vi "Update State Data.vi"(8 "error in (no error)":errorcluster, 9 "Data":variant, 10 "Argument":string, 11 "State Data":T1={"Core"={"Current VI Reference"=refnum, "Close Panel on Exit?"=FALSE}, "FP Refs"={"VI Tree"=refnum, "Window Title"=refnum, "Same Title as VI?"=refnum, "VI Desc"=refnum, "Help Path"=refnum, "Help Tag"=refnum, "Help URL"=refnum, "Controls"=refnum, "VI Connector Pane"=refnum, "Path to VI"=refnum, "Inlined?"=refnum, "Allow Debugging?"=refnum, "Auto Error Handling?"=refnum, "Run When Opened?"=refnum, "Suspend When Called?"=refnum, "Reentrancy"=refnum, "Priority"=refnum, "Preferred Exec System"=refnum, "VI Type"=refnum, "Edit Icon"=refnum, "Add Copyright"=refnum, "Set all VIs"=refnum, "Help Used"=refnum}, "Current Path"=path "", "New Item Data"=[], "Saved Item Data"=[], "FP"={"Selected VI Data"=0, "Help Path"="", "Help Tag"="", "Help URL"="", "Help Type"=enum."Local Help File", "VI Desc"="", "Controls"=[], "Window Title"="", "Same Title?"=FALSE, "VI Tree Value"=""}, "Config Path"=path "", "Config"={"ItemsEdited"=0, "Copyright Path"=path "", "Copyright Delimiter"="", "Recent Folders"=[], "Recent Files"=[], "Recent Filters"=[], "Abbreviate Names?"=FALSE, "Format Bold Tags?"=FALSE, "Show ConPane Only?"=FALSE, "Show Top-Level Only?"=FALSE, "Confirm Save?"=FALSE, "Confirm Revert?"=FALSE, "Confirm Save All?"=FALSE, "Confirm Revert All?"=FALSE, "Confirm Exit?"=FALSE, "Flat View?"=FALSE, "Ctls Sort Column"=0, "Ctls Sort Order"=0}, "Desc Selection"={"Selection Start"=0, "Selection End"=0}, "Displayed Indices"=[], "Filter"={"Filter Column"=enum."Description", "Filter Type"=enum."Contains", "Filter Value"="", "New Data?"=FALSE, "Case Sensitive?"=FALSE, "Enabled?"=FALSE}, "Sort"={"Sort Column"=enum."Description", "Ascending?"=FALSE, "Enabled?"=FALSE}, "Tree Map"=refnum, "Last Save Count"=0, "View Saved?"=FALSE, "Selected Item"=refnum}) -> (0 "error out":errorcluster, 3 "State Data out":T1={"Core"={"Current VI Reference"=refnum, "Close Panel on Exit?"=FALSE}, "FP Refs"={"VI Tree"=refnum, "Window Title"=refnum, "Same Title as VI?"=refnum, "VI Desc"=refnum, "Help Path"=refnum, "Help Tag"=refnum, "Help URL"=refnum, "Controls"=refnum, "VI Connector Pane"=refnum, "Path to VI"=refnum, "Inlined?"=refnum, "Allow Debugging?"=refnum, "Auto Error Handling?"=refnum, "Run When Opened?"=refnum, "Suspend When Called?"=refnum, "Reentrancy"=refnum, "Priority"=refnum, "Preferred Exec System"=refnum, "VI Type"=refnum, "Edit Icon"=refnum, "Add Copyright"=refnum, "Set all VIs"=refnum, "Help Used"=refnum}, "Current Path"=path "", "New Item Data"=[], "Saved Item Data"=[], "FP"={"Selected VI Data"=0, "Help Path"="", "Help Tag"="", "Help URL"="", "Help Type"=enum."Local Help File", "VI Desc"="", "Controls"=[], "Window Title"="", "Same Title?"=FALSE, "VI Tree Value"=""}, "Config Path"=path "", "Config"={"ItemsEdited"=0, "Copyright Path"=path "", "Copyright Delimiter"="", "Recent Folders"=[], "Recent Files"=[], "Recent Filters"=[], "Abbreviate Names?"=FALSE, "Format Bold Tags?"=FALSE, "Show ConPane Only?"=FALSE, "Show Top-Level Only?"=FALSE, "Confirm Save?"=FALSE, "Confirm Revert?"=FALSE, "Confirm Save All?"=FALSE, "Confirm Revert All?"=FALSE, "Confirm Exit?"=FALSE, "Flat View?"=FALSE, "Ctls Sort Column"=0, "Ctls Sort Order"=0}, "Desc Selection"={"Selection Start"=0, "Selection End"=0}, "Displayed Indices"=[], "Filter"={"Filter Column"=enum."Description", "Filter Type"=enum."Contains", "Filter Value"="", "New Data?"=FALSE, "Case Sensitive?"=FALSE, "Enabled?"=FALSE}, "Sort"={"Sort Column"=enum."Description", "Ascending?"=FALSE, "Enabled?"=FALSE}, "Tree Map"=refnum, "Last Save Count"=0, "View Saved?"=FALSE, "Selected Item"=refnum})   [LabVIEW 2020, in "VI Properties Editor.lvlib"]
doc: "Updates one or more elements of <B>State Data</B> based on <B>Argument</B> and <B>Data</B>."
uses:
  VI Properties Editor.lvlib
  Classes/Tree Map/Project Tree Map.lvclass
  Classes/Item/Item.lvclass
  Classes/VI/VI.lvclass
  <vilib>/ErrorRing/Error Ring.xnode
  Classes/Control/Control.lvclass
  3573416a-ab14-40fa-8eb1-e5c23e8662a1.vi
  6c3ab29c-e086-46da-822f-1f7a3bdde8cc.vi
  CTLs/Filter Column.ctl
  CTLs/Filter Type.ctl
  c05ae38d-f8ec-456d-8819-95a6d1f6576e.vi
  CTLs/Sort Column.ctl
  <vilib>/Utility/error.llb/Error Cluster From Error Code.vi
  CTLs/Main Front Panel Controls.ctl
  CTLs/Config.ctl
  <vilib>/Utility/miscctls.llb/LVSelectionTypeDef.ctl
  CTLs/Filter Info.ctl
  CTLs/Main References.ctl
  CTLs/Main State Data.ctl
  CTLs/Sort Info.ctl
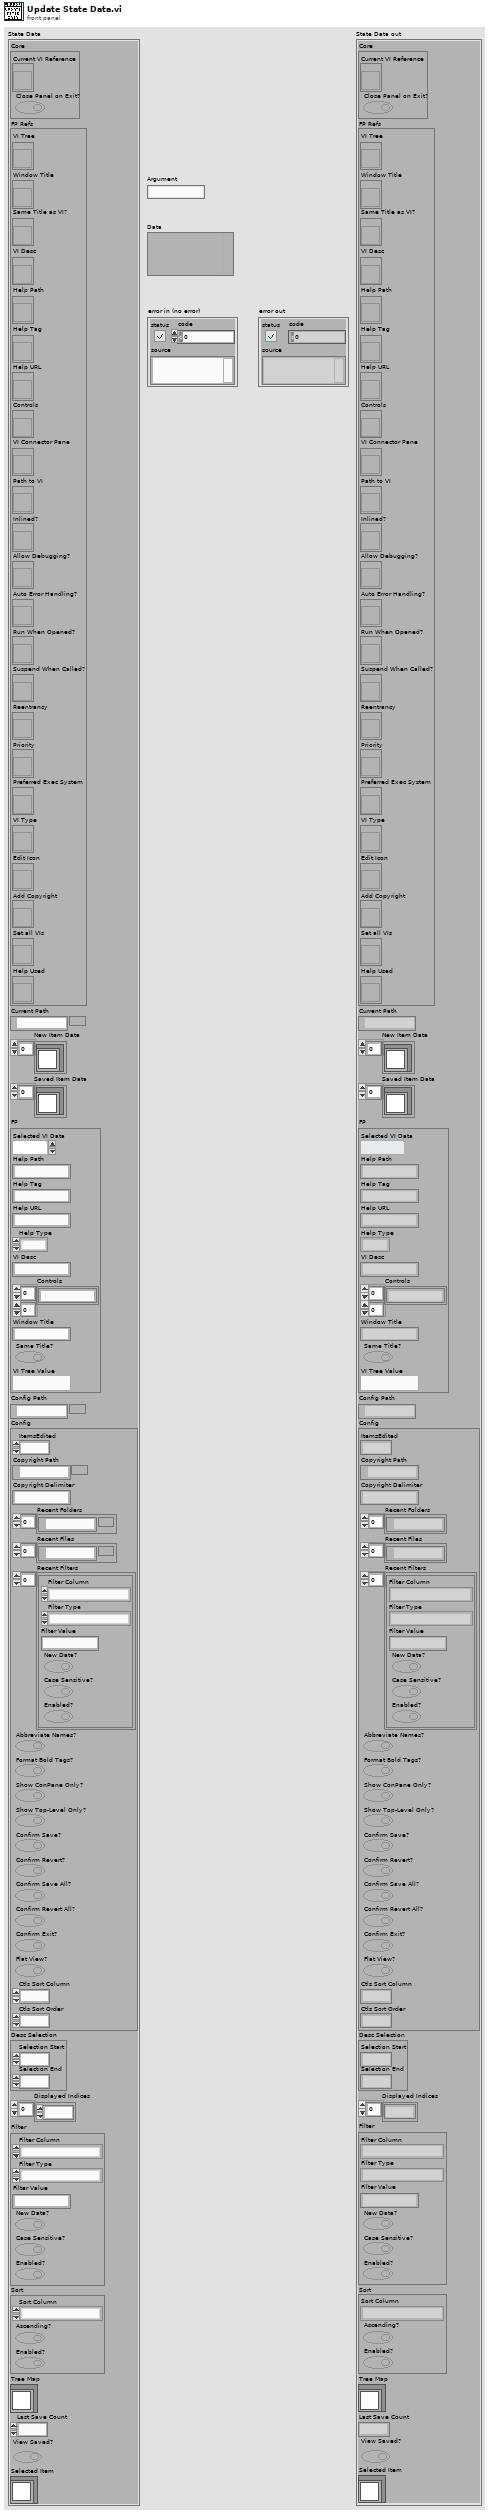
[diagram p1: front panel]
types:
  T1 = typedef "VI Properties Editor.lvlib/Main State Data.ctl" = cluster{"Core":cluster{"Current VI Reference":refnum<vi>, "Close Panel on Exit?":bool}, "FP Refs":T2, "Current Path":path, "New Item Data":refnum<class "Item.lvclass">[], "Saved Item Data":refnum<class "Item.lvclass">[], "FP":T3, "Config Path":path, "Config":T4, "Desc Selection":T8, "Displayed Indices":i32[], "Filter":T5, "Sort":T9, "Tree Map":refnum<class "Project Tree Map.lvclass">, "Last Save Count":u32, "View Saved?":bool, "Selected Item":refnum<class "Item.lvclass">}
  T2 = typedef "VI Properties Editor.lvlib/Main References.ctl" = cluster{"VI Tree":refnum<vi>, "Window Title":refnum<vi>, "Same Title as VI?":refnum<vi>, "VI Desc":refnum<vi>, "Help Path":refnum<vi>, "Help Tag":refnum<vi>, "Help URL":refnum<vi>, "Controls":refnum<vi>, "VI Connector Pane":refnum<vi>, "Path to VI":refnum<vi>, "Inlined?":refnum<vi>, "Allow Debugging?":refnum<vi>, "Auto Error Handling?":refnum<vi>, "Run When Opened?":refnum<vi>, "Suspend When Called?":refnum<vi>, "Reentrancy":refnum<vi>, "Priority":refnum<vi>, "Preferred Exec System":refnum<vi>, "VI Type":refnum<vi>, "Edit Icon":refnum<vi>, "Add Copyright":refnum<vi>, "Set all VIs":refnum<vi>, "Help Used":refnum<vi>}
  T3 = typedef "VI Properties Editor.lvlib/Main Front Panel Controls.ctl" = cluster{"Selected VI Data":i32, "Help Path":string, "Help Tag":string, "Help URL":string, "Help Type":enum16{"Local Help File", "Web-based Help"}, "VI Desc":string, "Controls":string[][], "Window Title":string, "Same Title?":bool, "VI Tree Value":string}
  T4 = typedef "VI Properties Editor.lvlib/Config.ctl" = cluster{"ItemsEdited":u32, "Copyright Path":path, "Copyright Delimiter":string, "Recent Folders":path[], "Recent Files":path[], "Recent Filters":T5[], "Abbreviate Names?":bool, "Format Bold Tags?":bool, "Show ConPane Only?":bool, "Show Top-Level Only?":bool, "Confirm Save?":bool, "Confirm Revert?":bool, "Confirm Save All?":bool, "Confirm Revert All?":bool, "Confirm Exit?":bool, "Flat View?":bool, "Ctls Sort Column":i32, "Ctls Sort Order":i32}
  T5 = typedef "VI Properties Editor.lvlib/Filter Info.ctl" = cluster{"Filter Column":T6, "Filter Type":T7, "Filter Value":string, "New Data?":bool, "Case Sensitive?":bool, "Enabled?":bool}
  T6 = typedef "VI Properties Editor.lvlib/Filter Column.ctl" = enum16{"Name", "Path", "Type", "Window Title", "Description", "Help Path", "Help Tag", "Custom Title?", "Reentrancy", "Inlined?", "Help URL", "Help Type", "Allow Debugging?", "Auto Error Handling?", "Run When Opened?", "Suspend When Called?", "Priority", "Preferred Exec Sytem", "Control Label", "Control Caption", "Control Description", "Control Tip Strip"}
  T7 = typedef "VI Properties Editor.lvlib/Filter Type.ctl" = enum16{"Contains", "Equals", "Starts with", "Ends with", "Is empty", "Does not contain", "Does not equal", "Is not empty"}
  T8 = typedef "LVSelectionTypeDef.ctl" = cluster{"Selection Start":u32, "Selection End":u32}
  T9 = typedef "VI Properties Editor.lvlib/Sort Info.ctl" = cluster{"Sort Column":T10, "Ascending?":bool, "Enabled?":bool}
  T10 = typedef "VI Properties Editor.lvlib/Sort Column.ctl" = enum16{"Name", "Filename", "Path", "Type", "Window Title", "Description", "Help Path", "Help Tag", "Custom Title?", "Reentrancy", "Inlined?", "Help URL", "Help Type", "Allow Debugging?", "Auto Error Handling?", "Run When Opened?", "Suspend When Called?", "Priority", "Preferred Exec Sytem"}
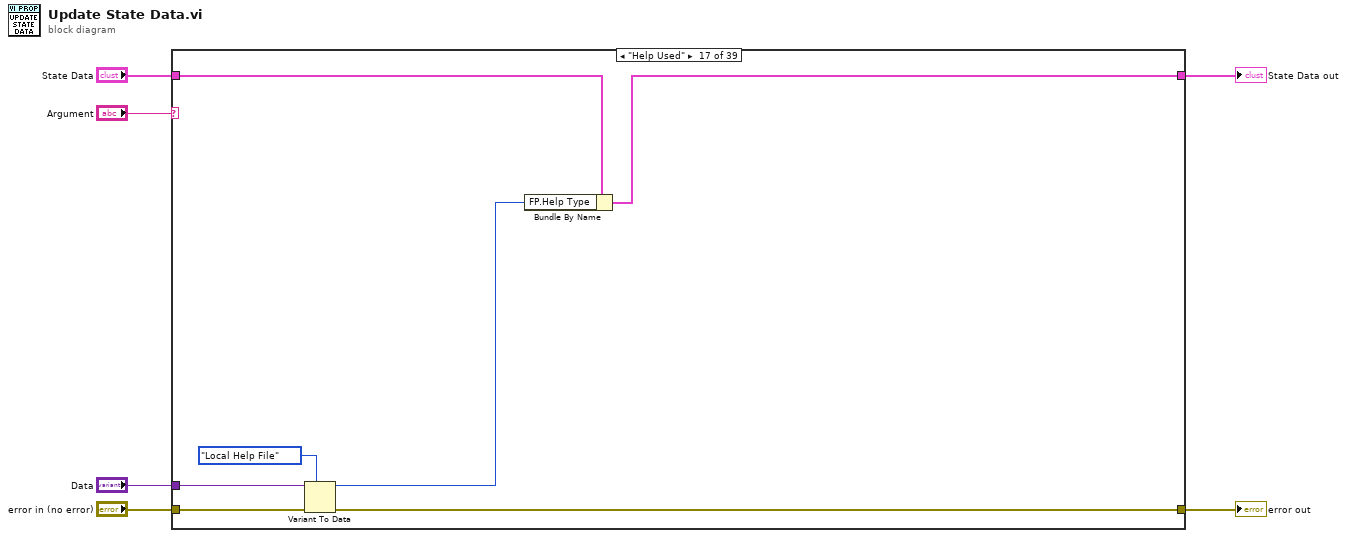
[diagram p0: block diagram]
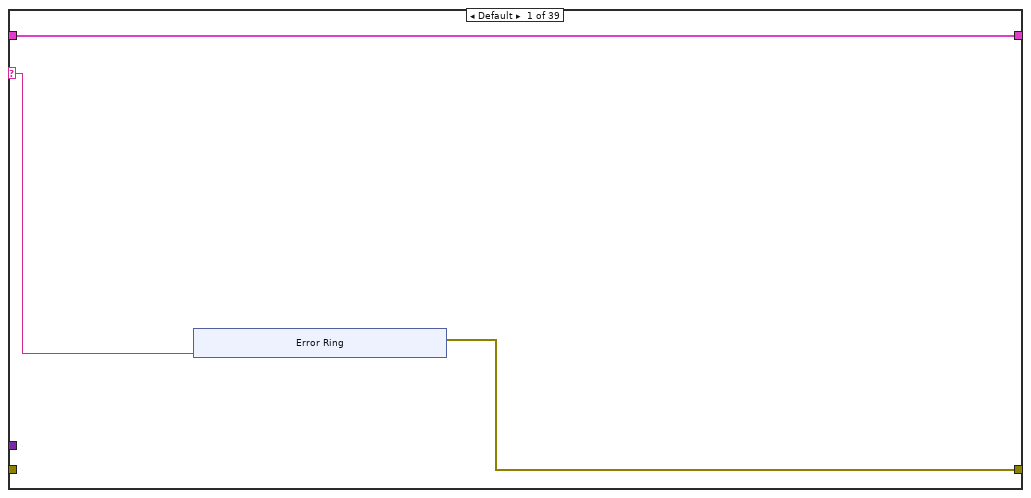
[diagram p2: hidden frame]
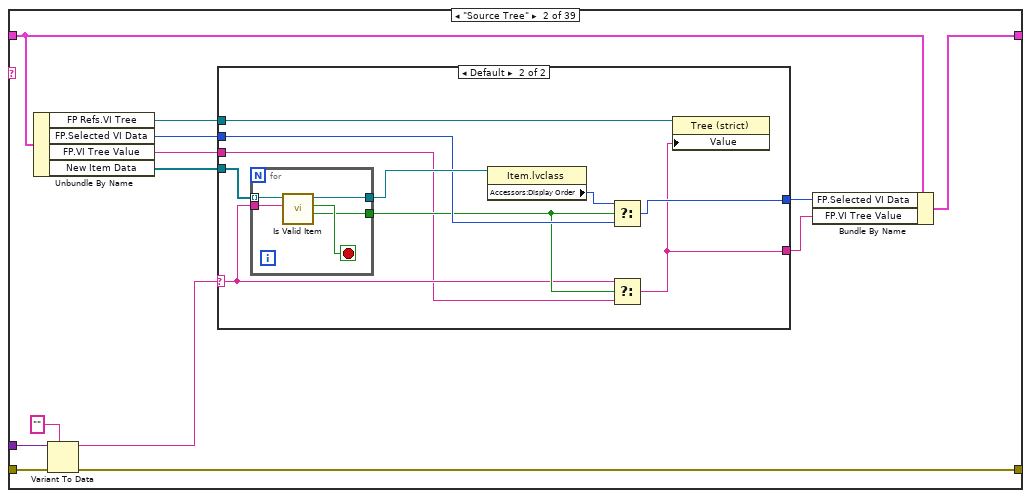
[diagram p3: hidden frame]
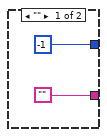
[diagram p4: hidden frame]
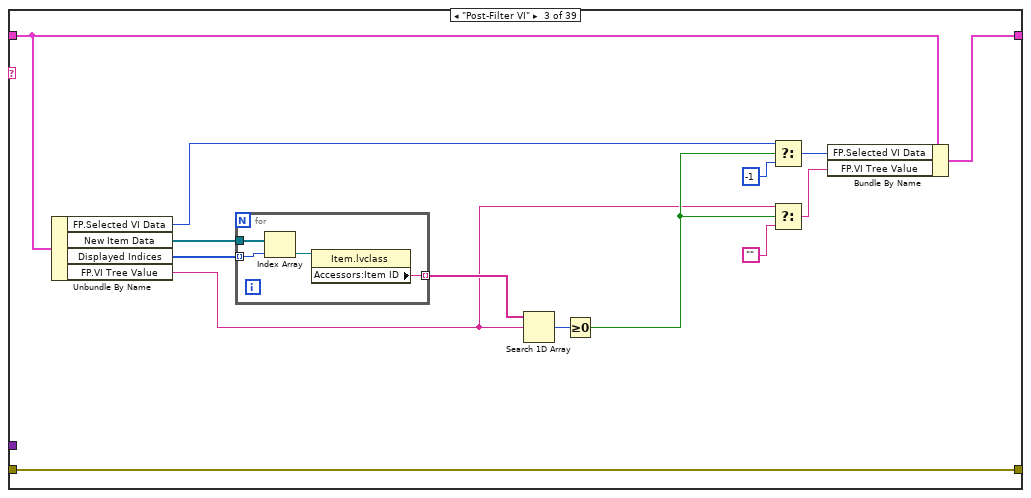
[diagram p5: hidden frame]
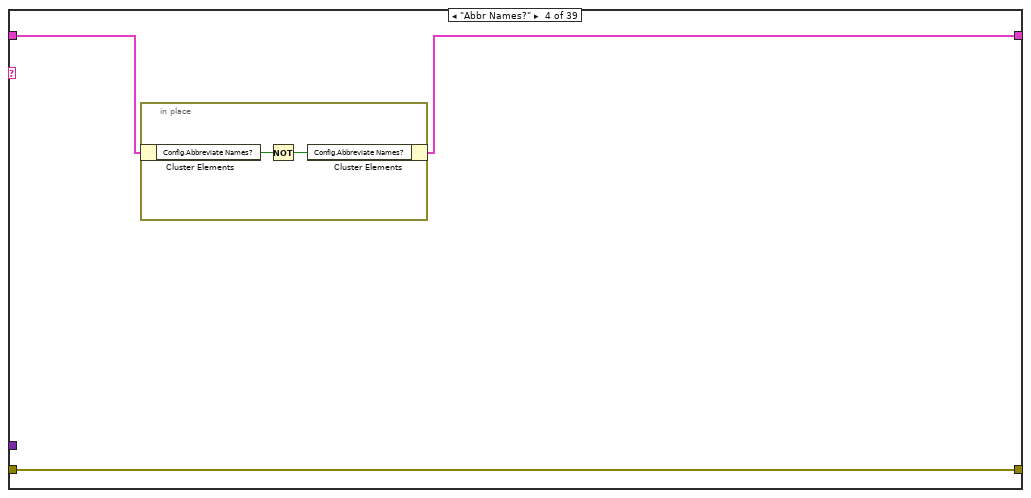
[diagram p6: hidden frame]
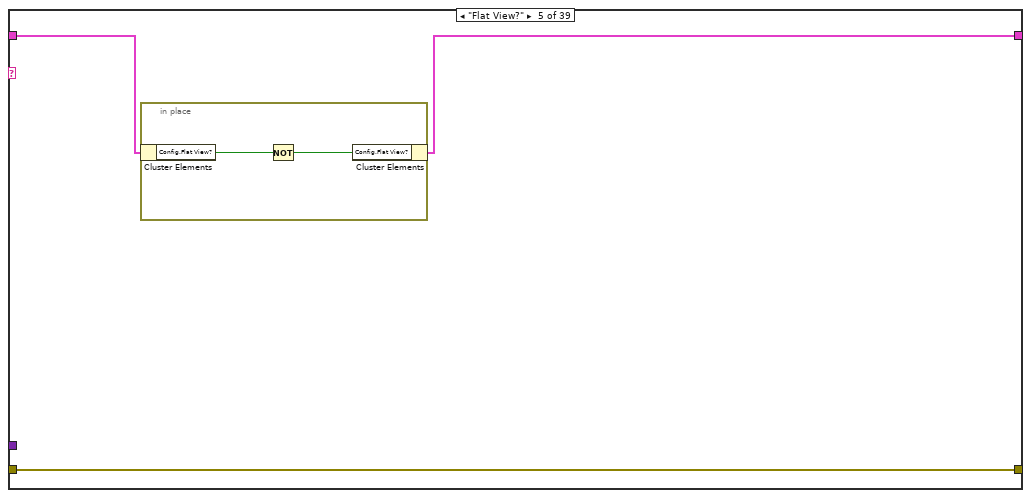
[diagram p7: hidden frame]
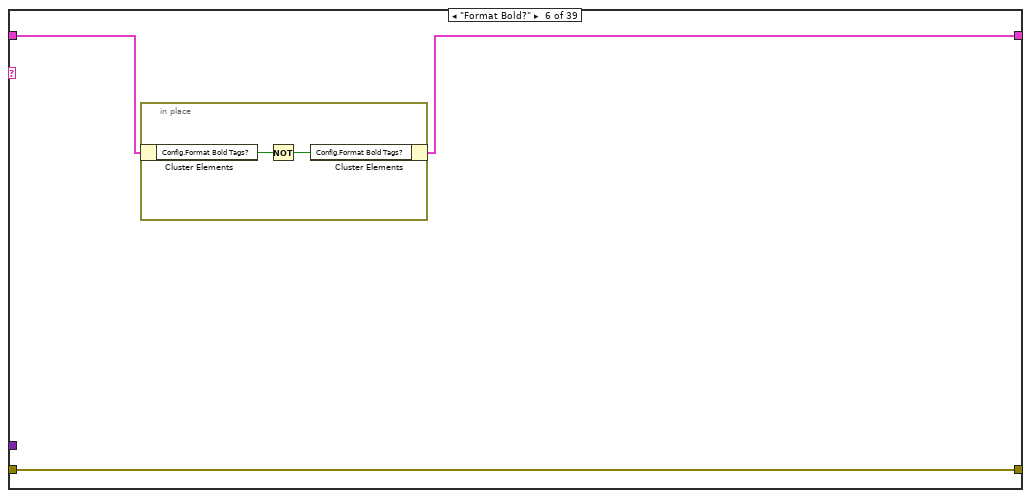
[diagram p8: hidden frame]
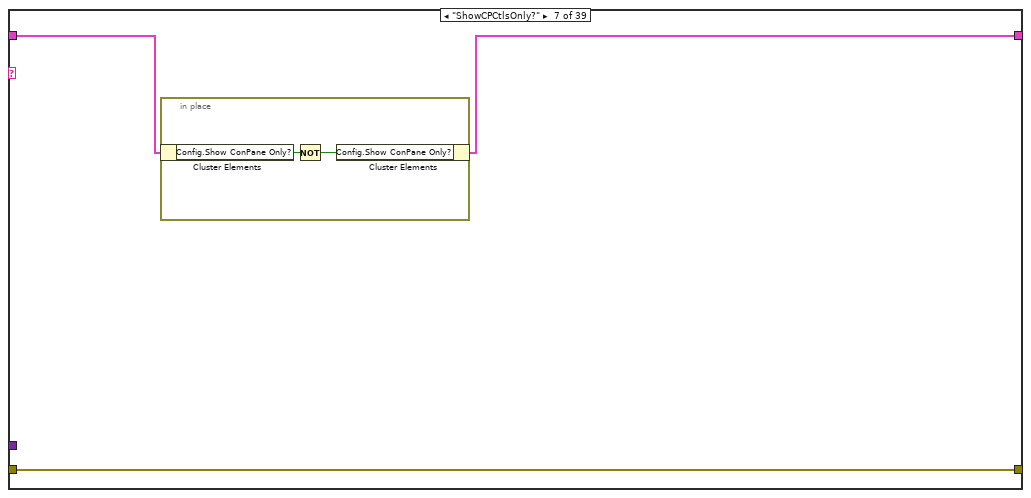
[diagram p9: hidden frame]
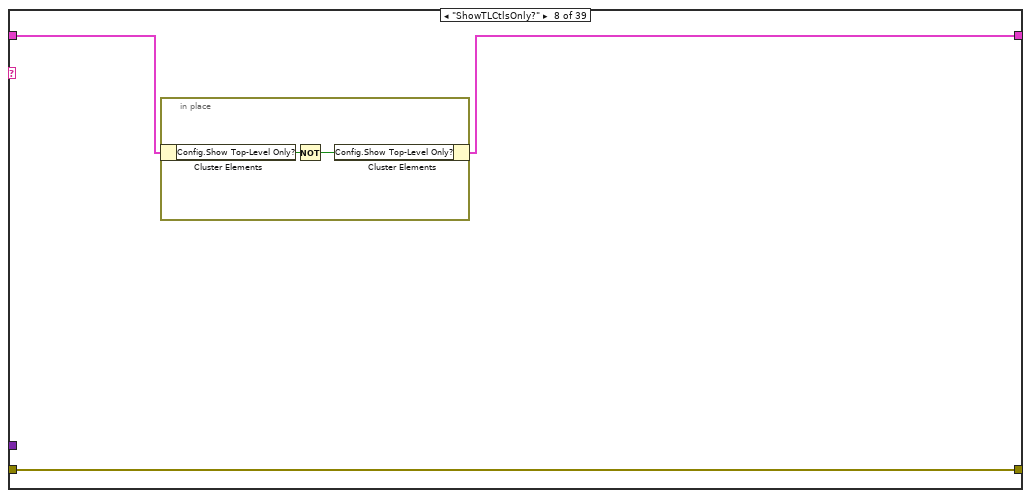
[diagram p10: hidden frame]
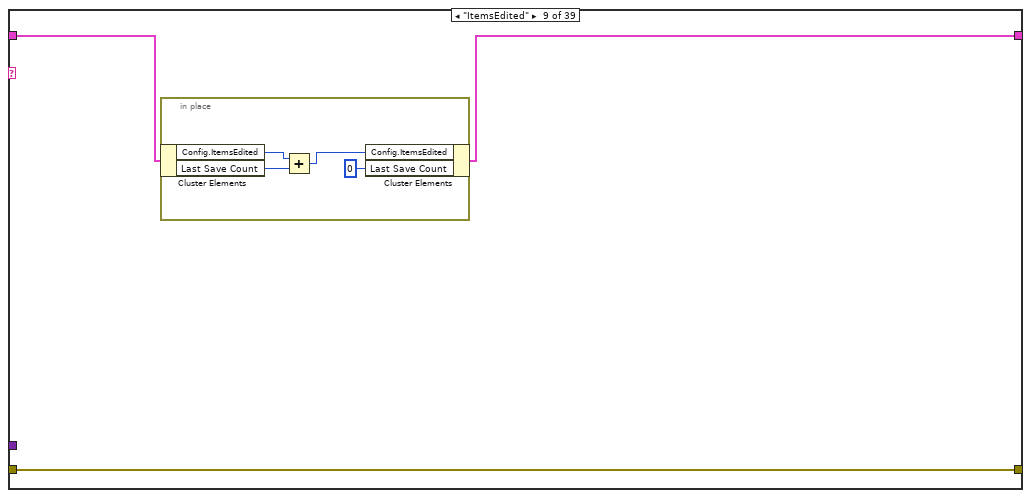
[diagram p11: hidden frame]
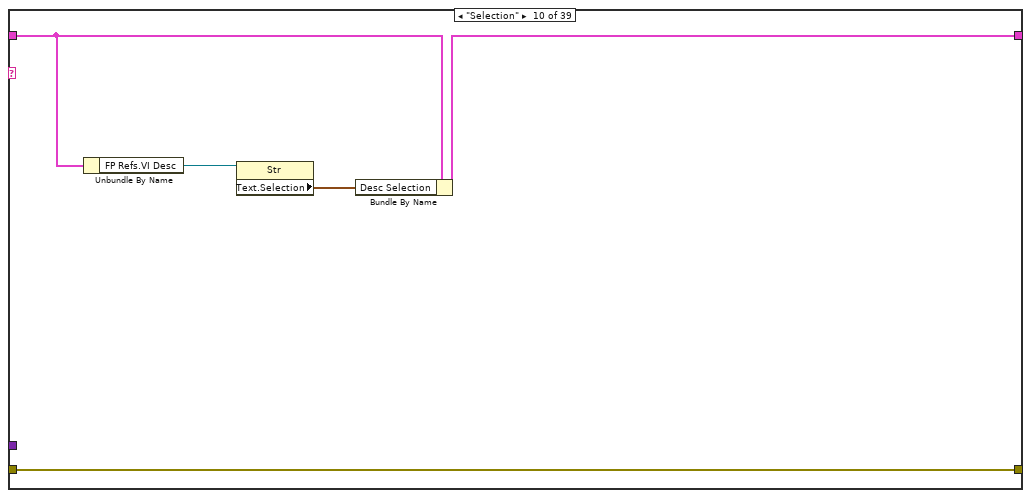
[diagram p12: hidden frame]
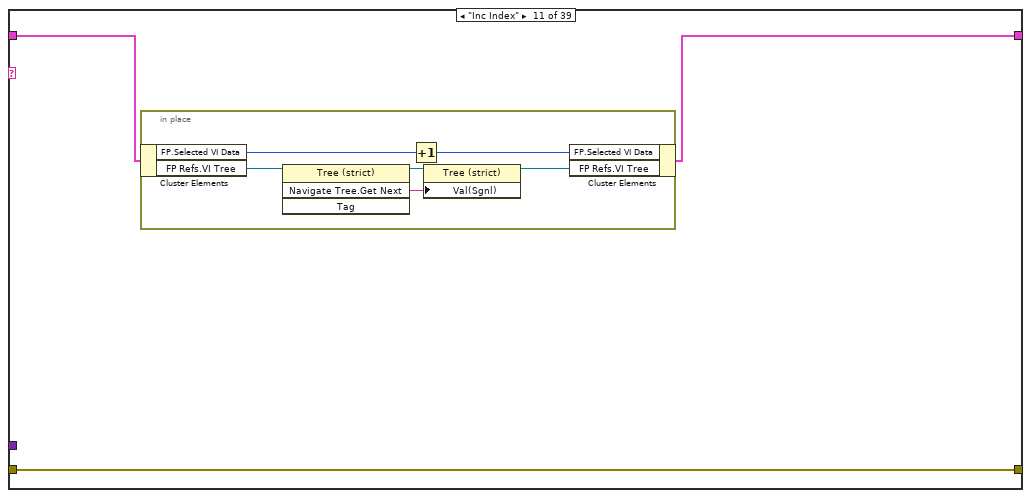
[diagram p13: hidden frame]
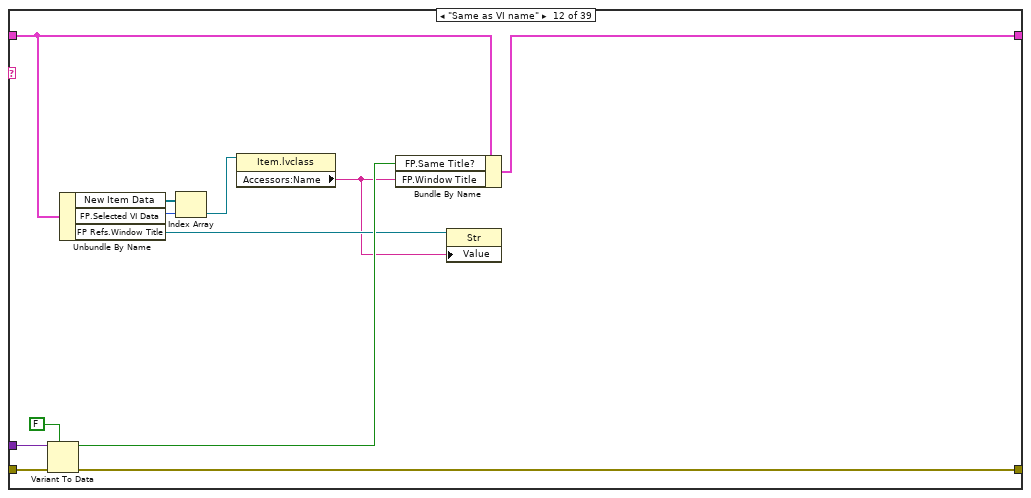
[diagram p14: hidden frame]
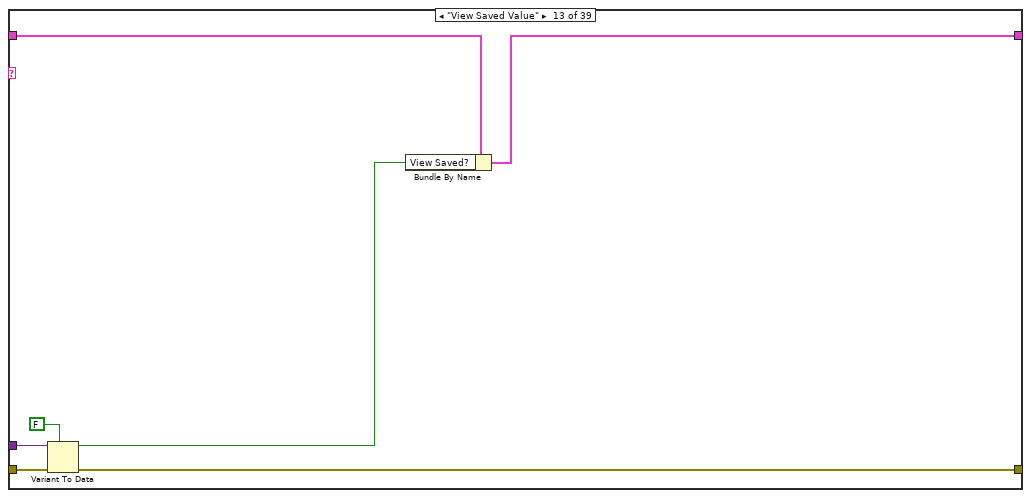
[diagram p15: hidden frame]
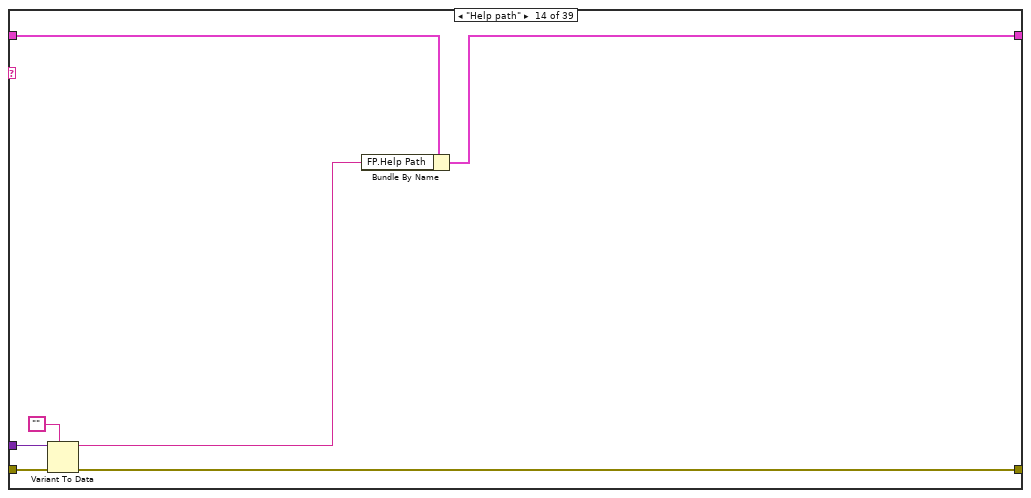
[diagram p16: hidden frame]
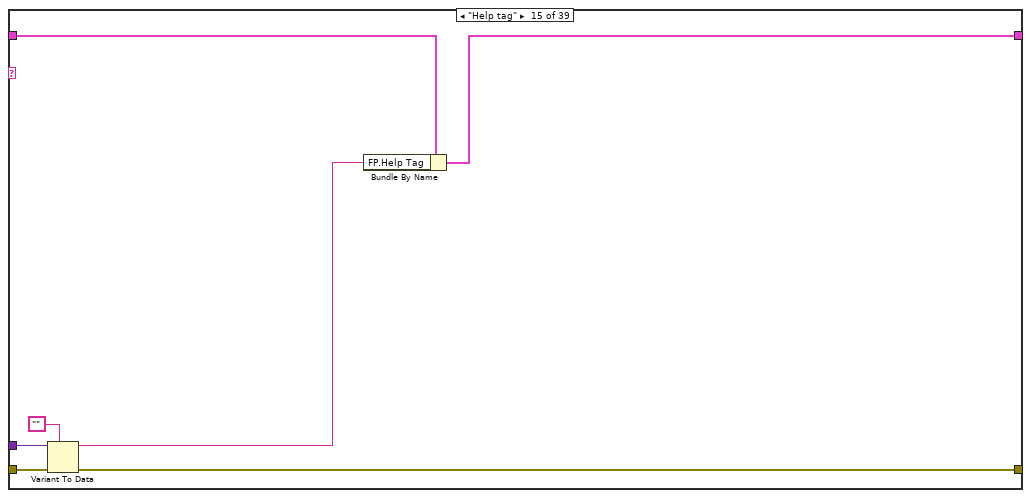
[diagram p17: hidden frame]
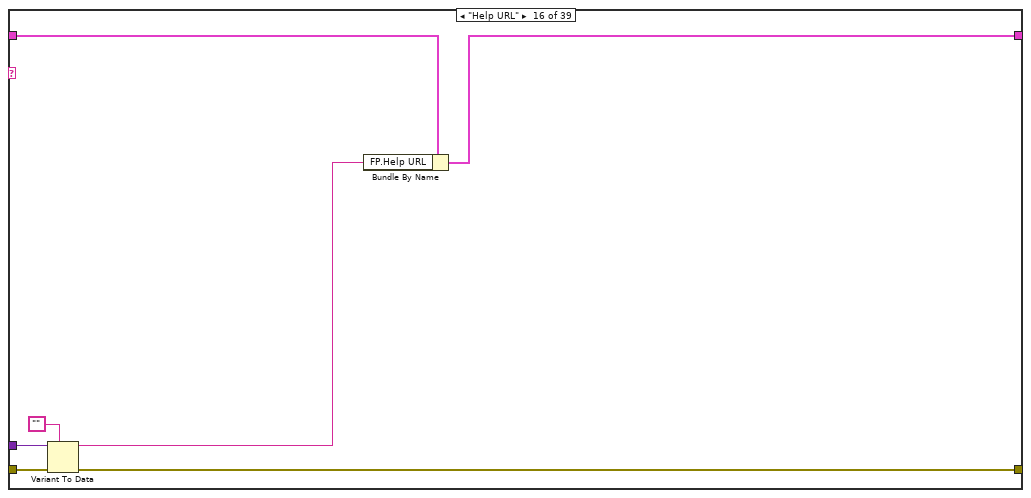
[diagram p18: hidden frame]
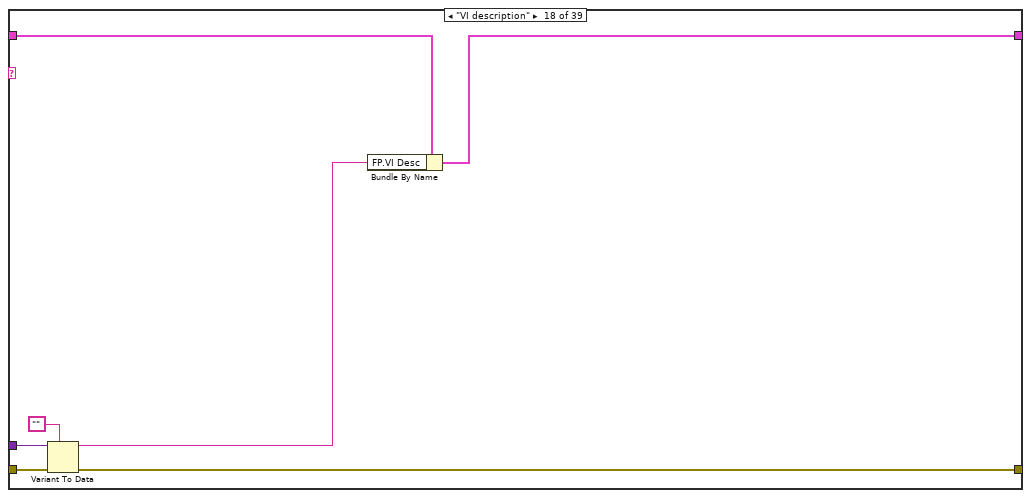
[diagram p19: hidden frame]
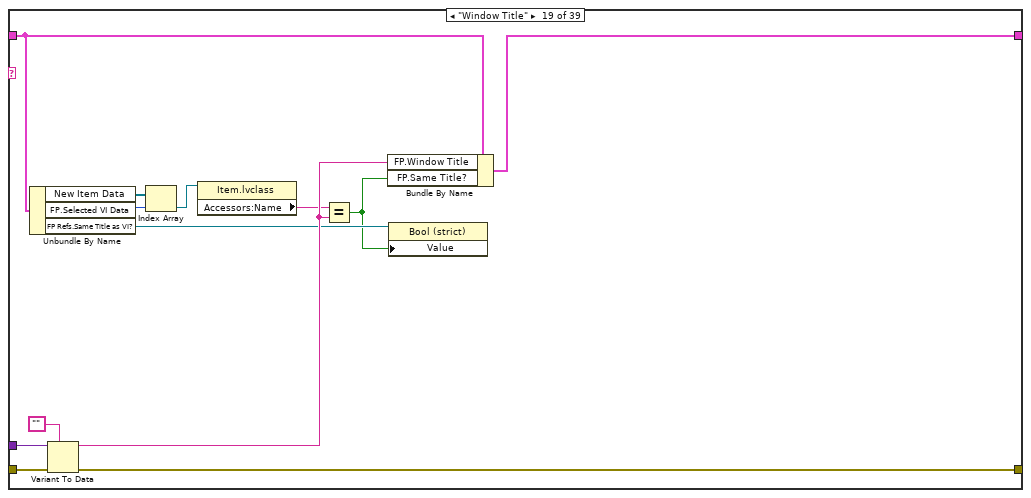
[diagram p20: hidden frame]
diagram:
  n1 = case shown="\"Help Used\"" "Argument" {
    selector: "Argument" -> [w8 _ _ _ _ _ _ _ _ _ _ _ _ _ _ _ _ _ _ _ _ _ _ _ _ w272 w282 w292 w307 w317 _ _ _ _ w352 _ _ _ _]
    tunnel: "error in (no error)" -> [_ w29 w58 w67 w72 w77 w82 w87 w92 w101 w104 w122 w129 w136 w143 w150 w157 w164 w177 w184 w217 w231 w241 w250 w259 w274 w284 w294 w309 w319 w325 w331 w338 w343 w354 w359 w364 w373 w384]
    tunnel: "State Data" -> [w9 w25 w59 w66 w71 w76 w81 w86 w91 w98 w103 w114 w123 w133 w140 w147 w155 w161 w170 w180 w221 w237 w239 w248 w257 w268 w278 w288 w303 w313 w323 w329 w336 w341 w349 w357 w362 w371 w382]
    tunnel: "Data" -> [_ w28 _ _ _ _ _ _ _ _ _ w121 w128 w135 w142 w149 w156 w163 w176 w183 _ _ _ _ _ _ _ _ _ _ _ _ _ _ _ _ _ w369 _]
    tunnel: [w7 w19 w58 w67 w72 w77 w82 w87 w92 w101 w104 w118 w125 w131 w138 w145 w154 w159 w174 w182 w216 w231 w241 w250 w259 w274 w284 w294 w309 w319 w325 w331 w338 w343 w354 w359 w364 w370 w384] -> w1
    tunnel: [w9 w26 w60 w65 w70 w75 w80 w85 w90 w99 w102 w117 w124 w130 w137 w144 w153 w158 w173 w178 w222 w238 w240 w249 w258 w273 w283 w293 w308 w318 w324 w330 w337 w342 w353 w358 w363 w372 w383] -> w5
    frame Default {
      n2 = xnode "Error Ring"("parameter 0"=w8) -> ("error out"=w7:errorcluster)
    }
    frame "Source Tree" {
      n3 = Unbundle By Name(w25) -> ("FP Refs.VI Tree"=w17:refnum<vi>, "FP.Selected VI Data"=w20:i32, "FP.VI Tree Value"=w21:string, "New Item Data"=w24:refnum<class "Item.lvclass">[])
      n4 = Variant To Data(error in=w29, type="", Variant=w28) -> (data=w18:string, error out=w19:errorcluster)
      n5 = case shown="Default" w18 {
        selector: w18 -> [_ w36]
        tunnel: w24 -> [_ w41]
        tunnel: [-1 w34] -> w23
        tunnel: ["" w32] -> w22
        tunnel: w21 -> [_ w35]
        tunnel: w20 -> [_ w38]
        tunnel: w17 -> [_ w33]
        frame "" {
        }
        frame Default {
          n6 = for {
            tunnel: w41 -> [w46] mode=indexing
            tunnel: w36 -> [w45]
            tunnel: [w43] -> w37
            tunnel: [w42] -> w40
            stop <- w44 stop-if-true
            n7 = call-dynamic "Is Valid Item.vi"("Item ID"=w45, "Item in"=w46) -> ("Is Valid?"=w43:bool, "Is Item?"=w44:bool, "Item out"=w42:refnum<class "Item.lvclass">)  [unwired: 6 in, 1 out]
          }
          n8 = property class="Item.lvclass"(reference=w40) -> ("Accessors:Display Order"=w39:i32)  [unwired: 1 in, 2 out]
          n9 = Select(t=w39, s=w37, f=w38) -> (s? t:f=w34:i32)
          n10 = Select(t=w36, s=w37, f=w35) -> (s? t:f=w32:string)
          n11 = property class="Tree (strict)"(reference=w33, "Value"=w32) -> ()  [unwired: 1 in, 2 out]
        }
      }
      n12 = Bundle By Name(cluster=w25, "FP.Selected VI Data"=w23, "FP.VI Tree Value"=w22) -> (w26:T1)
    }
    frame "Post-Filter VI" {
      n13 = Unbundle By Name(w59) -> ("FP.Selected VI Data"=w55:i32, "New Item Data"=w52:refnum<class "Item.lvclass">[], "Displayed Indices"=w51:i32[], "FP.VI Tree Value"=w47:string)
      n14 = for {
        tunnel: w52 -> [w63]
        tunnel: w51 -> [w64] mode=indexing
        tunnel: [w61] -> w50 mode=indexing
        n15 = Index Array(array=w63, index=w64) -> (element=w62:refnum<class "Item.lvclass">)
        n16 = property class="Item.lvclass"(reference=w62) -> ("Accessors:Item ID"=w61:string)  [unwired: 1 in, 2 out]
      }
      n17 = Search 1D Array(1D array=w50, element=w47) -> (index of element=w49:i32)  [unwired: 1 in]
      n18 = Greater Or Equal To 0?(x=w49) -> (x >= 0?=w48:bool)
      n19 = Select(t=w55, s=w48, f=-1) -> (s? t:f=w57:i32)
      n20 = Select(t=w47, s=w48, f="") -> (s? t:f=w54:string)
      n21 = Bundle By Name(cluster=w59, "FP.Selected VI Data"=w57, "FP.VI Tree Value"=w54) -> (w60:T1)
    }
    frame "Abbr Names?" {
      n22 = in-place {
        n23 = in-place-cluster #1(w66) -> ("Config.Abbreviate Names?"=w69:bool)
        n24 = Not(x=w69) -> (.not. x?=w68:bool)
        n25 = in-place-cluster #1("Config.Abbreviate Names?"=w68) -> (w65:T1)
      }
    }
    frame "Flat View?" {
      n26 = in-place {
        n27 = in-place-cluster #2(w71) -> ("Config.Flat View?"=w74:bool)
        n28 = Not(x=w74) -> (.not. x?=w73:bool)
        n29 = in-place-cluster #2("Config.Flat View?"=w73) -> (w70:T1)
      }
    }
    frame "Format Bold?" {
      n30 = in-place {
        n31 = in-place-cluster #3(w76) -> ("Config.Format Bold Tags?"=w79:bool)
        n32 = Not(x=w79) -> (.not. x?=w78:bool)
        n33 = in-place-cluster #3("Config.Format Bold Tags?"=w78) -> (w75:T1)
      }
    }
    frame "ShowCPCtlsOnly?" {
      n34 = in-place {
        n35 = in-place-cluster #4(w81) -> ("Config.Show ConPane Only?"=w84:bool)
        n36 = Not(x=w84) -> (.not. x?=w83:bool)
        n37 = in-place-cluster #4("Config.Show ConPane Only?"=w83) -> (w80:T1)
      }
    }
    frame "ShowTLCtlsOnly?" {
      n38 = in-place {
        n39 = in-place-cluster #5(w86) -> ("Config.Show Top-Level Only?"=w89:bool)
        n40 = Not(x=w89) -> (.not. x?=w88:bool)
        n41 = in-place-cluster #5("Config.Show Top-Level Only?"=w88) -> (w85:T1)
      }
    }
    frame "ItemsEdited" {
      n42 = in-place {
        n43 = in-place-cluster #6(w91) -> ("Config.ItemsEdited"=w96:u32, "Last Save Count"=w95:u32)
        n44 = Add(x=w96, y=w95) -> (x+y=w94:u32)
        n45 = in-place-cluster #6("Config.ItemsEdited"=w94, "Last Save Count"=u32 0) -> (w90:T1)
      }
    }
    frame "Selection" {
      n46 = Unbundle By Name(w98) -> ("FP Refs.VI Desc"=w97:refnum<vi>)
      n47 = property on="Property Node" class="Str"(reference=w97) -> ("Text.Selection"=w100:T8)  [unwired: 1 in, 2 out]
      n48 = Bundle By Name(cluster=w98, "Desc Selection"=w100) -> (w99:T1)
    }
    frame "Inc Index" {
      n49 = in-place {
        n50 = in-place-cluster #7(w103) -> ("FP.Selected VI Data"=w110:i32, "FP Refs.VI Tree"=w109:refnum<vi>)
        n51 = invoke class="Tree (strict)" method="Navigate Tree.Get Next"(reference=w109) -> (reference out=w108:refnum<vi>, "Navigate Tree:Get Next Item"=w105:string)  [unwired: 3 in, 2 out]
        n52 = Increment(x=w110) -> (x+1=w107:i32)
        n53 = property class="Tree (strict)"(reference=w108, "Val(Sgnl)"=w105) -> (reference out=w106:refnum<vi>)  [unwired: 1 in, 1 out]
        n54 = in-place-cluster #7("FP.Selected VI Data"=w107, "FP Refs.VI Tree"=w106) -> (w102:T1)
      }
    }
    frame "Same as VI name" {
      n55 = Variant To Data(error in=w122, type=FALSE, Variant=w121) -> (data=w119:bool, error out=w118:errorcluster)
      n56 = Unbundle By Name(w114) -> ("New Item Data"=w116:refnum<class "Item.lvclass">[], "FP.Selected VI Data"=w115:i32, "FP Refs.Window Title"=w113:refnum<vi>)
      n57 = Index Array(array=w116, index=w115) -> (element=w112:refnum<class "Item.lvclass">)
      n58 = property class="Item.lvclass"(reference=w112) -> ("Accessors:Name"=w111:string)  [unwired: 1 in, 2 out]
      n59 = Bundle By Name(cluster=w114, "FP.Same Title?"=w119, "FP.Window Title"=w111) -> (w117:T1)
      n60 = property class="Str"(reference=w113, "Value"=w111) -> ()  [unwired: 1 in, 2 out]
    }
    frame "View Saved Value" {
      n61 = Variant To Data(error in=w129, type=FALSE, Variant=w128) -> (data=w126:bool, error out=w125:errorcluster)
      n62 = Bundle By Name(cluster=w123, "View Saved?"=w126) -> (w124:T1)
    }
    frame "Help path" {
      n63 = Variant To Data(error in=w136, type="", Variant=w135) -> (data=w132:string, error out=w131:errorcluster)
      n64 = Bundle By Name(cluster=w133, "FP.Help Path"=w132) -> (w130:T1)
    }
    frame "Help tag" {
      n65 = Variant To Data(error in=w143, type="", Variant=w142) -> (data=w139:string, error out=w138:errorcluster)
      n66 = Bundle By Name(cluster=w140, "FP.Help Tag"=w139) -> (w137:T1)
    }
    frame "Help URL" {
      n67 = Variant To Data(error in=w150, type="", Variant=w149) -> (data=w146:string, error out=w145:errorcluster)
      n68 = Bundle By Name(cluster=w147, "FP.Help URL"=w146) -> (w144:T1)
    }
    frame "Help Used" {
      n69 = Variant To Data(error in=w157, type=enum16{"Local Help File", "Web-based Help"}."Local Help File" ("FP.Help Type"), Variant=w156) -> (data=w151:enum16{"Local Help File", "Web-based Help"}, error out=w154:errorcluster)
      n70 = Bundle By Name(cluster=w155, "FP.Help Type"=w151) -> (w153:T1)
    }
    frame "VI description" {
      n71 = Variant To Data(error in=w164, type="", Variant=w163) -> (data=w160:string, error out=w159:errorcluster)
      n72 = Bundle By Name(cluster=w161, "FP.VI Desc"=w160) -> (w158:T1)
    }
    frame "Window Title" {
      n73 = Unbundle By Name(w170) -> ("New Item Data"=w172:refnum<class "Item.lvclass">[], "FP.Selected VI Data"=w171:i32, "FP Refs.Same Title as VI?"=w168:refnum<vi>)
      n74 = Variant To Data(error in=w177, type="", Variant=w176) -> (data=w169:string, error out=w174:errorcluster)
      n75 = Index Array(array=w172, index=w171) -> (element=w166:refnum<class "Item.lvclass">)
      n76 = property class="Item.lvclass"(reference=w166) -> ("Accessors:Name"=w165:string)  [unwired: 1 in, 2 out]
      n77 = Equal?(x=w165, y=w169) -> (x = y?=w167:bool)
      n78 = Bundle By Name(cluster=w170, "FP.Window Title"=w169, "FP.Same Title?"=w167) -> (w173:T1)
      n79 = property class="Bool (strict)"(reference=w168, "Value"=w167) -> ()  [unwired: 1 in, 2 out]
    }
    frame "Controls" {
      n80 = Variant To Data(error in=w184, type=string[][] [], Variant=w183) -> (data=w179:string[][], error out=w182:errorcluster)
      n81 = in-place {
        in-place-border: w179 -> [w200]
        # "Only keep label, caption, description, and tip strip field changes"
        n82 = in-place-cluster #8(w180) -> ("FP Refs.Controls"=w189:refnum<vi>, "FP.Controls"=w199:string[][])
        n83 = Index Array(array=w200, index (col) #1=0 ("disabled index (col)"), index (col) #2=2 ("index (row)"), index (col) #3=3 ("index (row)"), index (col) #4=4 ("index (row)")) -> (element #1=w192:string[], element #2=w191:string[], element #3=w190:string[], element #4=w185:string[])  [unwired: 4 in]
        n84 = Replace Array Subset(array=w199, new element #1=w192, index (col) #1=0 ("index (row)"), new element #2=w191, index (col) #2=2 ("index (row)"), new element #3=w190, index (col) #3=3 ("index (row)"), new element #4=w185, index (col) #4=4 ("index (row)")) -> (w187:string[][])  [unwired: 4 in]
        n85 = property class="Tbl (strict)"(reference=w189, "Value"=w187) -> (reference out=w188:refnum<vi>)  [unwired: 1 in, 1 out]
        n86 = in-place-cluster #8("FP Refs.Controls"=w188, "FP.Controls"=w187) -> (w178:T1)
      }
    }
    frame "All Ctls" {
      # "Handles the case of index being out of array size"
      n87 = Unbundle By Name(w221) -> ("Config.Show ConPane Only?"=w205:bool, "Config.Show Top-Level Only?"=w206:bool, "Config.Ctls Sort Column"=w203:i32, "Config.Ctls Sort Order"=w202:i32, "Selected Item"=w204:refnum<class "Item.lvclass">)
      n88 = Not Equal?(x=refnum<class "Item.lvclass"> refnum ("element"), y=w204) -> (x != y?=w207:bool)
      n89 = case shown="True" w207 {
        tunnel: w204 -> [_ w229]
        tunnel: w217 -> [w224 w227]
        tunnel: [w224 w226] -> w216
        tunnel: [refnum<class "VI.lvclass"> refnum ("VI Properties Editor.lvlib:VI.lvclass") w225] -> w215
        frame False {
        }
        frame True {
          n90 = To More Specific Class(target class=refnum<class "VI.lvclass"> refnum ("VI Properties Editor.lvlib:VI.lvclass"), reference=w229, error in=w227) -> (specific class reference=w225:refnum<class "VI.lvclass">, error out=w226:errorcluster)
        }
      }
      n91 = property class="VI.lvclass"(reference=w215) -> ("Accessors:Controls Data"=w209:refnum<class "Control.lvclass">[], "Accessors:Help Tag"=w210:string, "Accessors:Help Path"=w211:path, "Accessors:Description"=w212:string, "Accessors:Window Title"=w213:string, "Accessors:Custom Title_"=w214:bool)  [unwired: 1 in, 2 out]
      n92 = call "Convert Controls to Arrays.vi"("Sort Order"=w202, "Sort Column"=w203, "Top-Level Only?"=w206, "ConPane Only?"=w205, "Controls Data"=w209) -> ("Control Array"=w220:string[][])  [unwired: 6 in]
      n93 = Path To String(path=w211) -> (string=w219:string)
      n94 = Not(x=w214) -> (.not. x?=w218:bool)
      n95 = Bundle By Name(cluster=w221, "FP.Controls"=w220, "FP.Help Tag"=w210, "FP.Help Path"=w219, "FP.VI Desc"=w212, "FP.Window Title"=w213, "FP.Same Title?"=w218) -> (w222:T1)
    }
    frame "Selected Item" {
      n96 = Unbundle By Name(w237) -> ("Saved Item Data"=w234:refnum<class "Item.lvclass">[], "View Saved?"=w235:bool, "New Item Data"=w233:refnum<class "Item.lvclass">[], "FP.Selected VI Data"=w236:i32)
      n97 = Select(t=w234, s=w235, f=w233) -> (s? t:f=w232:refnum<class "Item.lvclass">[])
      n98 = Index Array(array=w232, index=w236) -> (element=w230:refnum<class "Item.lvclass">)
      n99 = Bundle By Name(cluster=w237, "Selected Item"=w230) -> (w238:T1)
    }
    frame "Folder Config" {
      n100 = in-place {
        n101 = in-place-cluster #9(w239) -> ("Current Path"=w244:path, "Config.Recent Folders"=w247:path[])
        n102 = Build Array (concatenate)(w244, w247) -> (w246:path[])
        n103 = Array Subset(array=w246, length=10) -> (w243:path[])  [unwired: 1 in]
        n104 = call "Remove Duplicates From 1D Array.vim"("array"=w243) -> ("array with duplicates removed"=w242:path[])  [unwired: 10 in]
        n105 = in-place-cluster #9("Current Path"=w244, "Config.Recent Folders"=w242) -> (w240:T1)
      }
    }
    frame "File Config" {
      n106 = in-place {
        n107 = in-place-cluster #10(w248) -> ("Current Path"=w253:path, "Config.Recent Files"=w256:path[])
        n108 = Build Array (concatenate)(w253, w256) -> (w255:path[])
        n109 = Array Subset(array=w255, length=10) -> (w252:path[])  [unwired: 1 in]
        n110 = call "Remove Duplicates From 1D Array.vim"("array"=w252) -> ("array with duplicates removed"=w251:path[])  [unwired: 10 in]
        n111 = in-place-cluster #10("Current Path"=w253, "Config.Recent Files"=w251) -> (w249:T1)
      }
    }
    frame "Filter Config" {
      n112 = in-place {
        # "don't want multiple of the same filter because one was filtered on new data"
        n113 = in-place-cluster #11(w257) -> ("Filter"=w262:T5, "Config.Recent Filters"=w267:T5[])
        n114 = Bundle By Name(cluster=w262, "New Data?"=FALSE) -> (w260:T5)
        n115 = Build Array (concatenate)(w260, w267) -> (w266:T5[])
        n116 = Array Subset(array=w266, length=10) -> (w264:T5[])  [unwired: 1 in]
        n117 = call "Remove Duplicates From 1D Array.vim"("array"=w264) -> ("array with duplicates removed"=w263:T5[])  [unwired: 10 in]
        n118 = in-place-cluster #11("Filter"=w262, "Config.Recent Filters"=w263) -> (w258:T1)
      }
    }
    frame "FOLDER_0".."FOLDER_9" {
      n119 = Match Pattern(string=w272, regular expression="_") -> (after substring=w270:string)  [unwired: 1 in, 3 out]
      n120 = Decimal String To Number(string=w270) -> (number=w269:i32)  [unwired: 2 in, 1 out]
      n121 = in-place {
        in-place-border: w269 -> [w276]
        n122 = in-place-cluster #12(w268) -> ("Config.Recent Folders"=w277:path[])  [unwired: 1 out]
        n123 = Index Array(array=w277, index=w276) -> (element=w275:path)
        n124 = in-place-cluster #12("Current Path"=w275, "Config.Recent Folders"=w277) -> (w273:T1)
      }
    }
    frame "FILE_0".."FILE_9" {
      n125 = Match Pattern(string=w282, regular expression="_") -> (after substring=w280:string)  [unwired: 1 in, 3 out]
      n126 = Decimal String To Number(string=w280) -> (number=w279:i32)  [unwired: 2 in, 1 out]
      n127 = in-place {
        in-place-border: w279 -> [w286]
        n128 = in-place-cluster #13(w278) -> ("Config.Recent Files"=w287:path[])  [unwired: 1 out]
        n129 = Index Array(array=w287, index=w286) -> (element=w285:path)
        n130 = in-place-cluster #13("Current Path"=w285, "Config.Recent Files"=w287) -> (w283:T1)
      }
    }
    frame "FILTER_0".."FILTER_9" {
      n131 = Match Pattern(string=w292, regular expression="_") -> (after substring=w290:string)  [unwired: 1 in, 3 out]
      n132 = Decimal String To Number(string=w290) -> (number=w289:i32)  [unwired: 2 in, 1 out]
      n133 = in-place {
        in-place-border: w289 -> [w301]
        n134 = in-place-cluster #14(w288) -> ("Config.Recent Filters"=w302:T5[])  [unwired: 5 out]
        n135 = Index Array(array=w302, index=w301) -> (element=w300:T5)
        n136 = Unbundle By Name(w300) -> ("Filter Column"=w299:T6, "Filter Type"=w298:T7, "Filter Value"=w297:string, "Case Sensitive?"=w295:bool)
        n137 = in-place-cluster #14("Config.Recent Filters"=w302, "Filter.Filter Column"=w299, "Filter.Filter Type"=w298, "Filter.Filter Value"=w297, "Filter.Case Sensitive?"=w295, "Filter.Enabled?"=TRUE) -> (w293:T1)
      }
    }
    frame "REM-FOLDER_0".."REM-FOLDER_9" {
      n138 = Match Pattern(string=w307, regular expression="_") -> (after substring=w305:string)  [unwired: 1 in, 3 out]
      n139 = Decimal String To Number(string=w305) -> (number=w304:i32)  [unwired: 2 in, 1 out]
      n140 = in-place {
        in-place-border: w304 -> [w311]
        n141 = in-place-cluster #15(w303) -> ("Config.Recent Folders"=w312:path[])
        n142 = Delete From Array(array=w312, index=w311) -> (array with subset deleted=w310:path[])  [unwired: 1 in, 1 out]
        n143 = in-place-cluster #15("Config.Recent Folders"=w310) -> (w308:T1)
      }
    }
    frame "REM-FILE_0".."REM-FILE_9" {
      n144 = Match Pattern(string=w317, regular expression="_") -> (after substring=w315:string)  [unwired: 1 in, 3 out]
      n145 = Decimal String To Number(string=w315) -> (number=w314:i32)  [unwired: 2 in, 1 out]
      n146 = in-place {
        in-place-border: w314 -> [w321]
        n147 = in-place-cluster #16(w313) -> ("Config.Recent Files"=w322:path[])
        n148 = Delete From Array(array=w322, index=w321) -> (array with subset deleted=w320:path[])  [unwired: 1 in, 1 out]
        n149 = in-place-cluster #16("Config.Recent Files"=w320) -> (w318:T1)
      }
    }
    frame "Filter" {
      n150 = in-place {
        n151 = in-place-cluster #17(w323) -> ()  [unwired: 3 out]
        n152 = in-place-cluster #17("Filter.Filter Column"=Filter_Column."Description", "Filter.Filter Type"=Filter_Type."Is empty", "Filter.Enabled?"=TRUE) -> (w324:T1)
      }
    }
    frame "Filter 2" {
      n153 = in-place {
        n154 = in-place-cluster #18(w329) -> ()  [unwired: 4 out]
        n155 = in-place-cluster #18("Filter.Filter Value"="<[Bb]>.+</[Bb]>", "Filter.Filter Column"=Filter_Column."Description", "Filter.Filter Type"=Filter_Type."Does not contain", "Filter.Enabled?"=TRUE) -> (w330:T1)
      }
    }
    frame "Filter Data Source" {
      n156 = in-place {
        n157 = in-place-cluster #19(w336) -> ("Filter.New Data?"=w340:bool)
        n158 = Not(x=w340) -> (.not. x?=w339:bool)
        n159 = in-place-cluster #19("Filter.New Data?"=w339) -> (w337:T1)
      }
    }
    frame "Clear Filter" {
      n160 = in-place {
        n161 = in-place-cluster #20(w341) -> ()  [unwired: 1 out]
        n162 = in-place-cluster #20("Filter.Enabled?"=FALSE) -> (w342:T1)
      }
    }
    frame "SORT_0".."SORT_99" {
      n163 = Match Pattern(string=w352, regular expression="_") -> (after substring=w350:string)  [unwired: 1 in, 3 out]
      n164 = Decimal String To Number(string=w350, default (0L)=u16 0 ("default (0 I32)")) -> (number=w348:u16)  [unwired: 1 in, 1 out]
      n165 = Type Cast(type=Sort_Column."Name" ("Sort.Sort Column"), x=w348) -> (*(type *) &x=w347:T10)
      n166 = in-place {
        in-place-border: w347 -> [w356]
        n167 = in-place-cluster #21(w349) -> ()  [unwired: 2 out]
        n168 = in-place-cluster #21("Sort.Enabled?"=TRUE, "Sort.Sort Column"=w356) -> (w353:T1)
      }
    }
    frame "Unsort" {
      n169 = in-place {
        n170 = in-place-cluster #22(w357) -> ()  [unwired: 2 out]
        n171 = in-place-cluster #22("Sort.Sort Column"=Sort_Column."Name", "Sort.Enabled?"=FALSE) -> (w358:T1)
      }
    }
    frame "Sort Order" {
      n172 = in-place {
        n173 = in-place-cluster #23(w362) -> ("Sort.Ascending?"=w366:bool)
        n174 = Not(x=w366) -> (.not. x?=w365:bool)
        n175 = in-place-cluster #23("Sort.Ascending?"=w365) -> (w363:T1)
      }
    }
    frame "Sort Column" {
      n176 = Variant To Data(error in=w373, type=0, Variant=w369) -> (data=w367:i32, error out=w370:errorcluster)
      n177 = in-place {
        in-place-border: w367 -> [w380]
        n178 = in-place-cluster #24(w371) -> ("Config.Ctls Sort Column"=w381:i32, "Config.Ctls Sort Order"=w376:i32)
        n179 = Equal?(x=w381, y=w380) -> (x = y?=w379:bool)
        n180 = Equal To 0?(x=w376) -> (x = 0?=w374:bool)
        n181 = Boolean To (0,1)(Boolean=w374) -> (0, 1=w375:i16)
        n182 = Select(t=w375, s=w379, f=0) -> (s? t:f=w377:i32)
        n183 = in-place-cluster #24("Config.Ctls Sort Column"=w380, "Config.Ctls Sort Order"=w377) -> (w372:T1)
      }
    }
    frame "Reset VI Tree" {
      n184 = in-place {
        n185 = in-place-cluster #25(w382) -> ("FP Refs.VI Tree"=w388:refnum<vi>)  [unwired: 2 out]
        n186 = invoke class="Tree (strict)" method="Edit Tree Items.Delete"(reference=w388) -> (reference out=w387:refnum<vi>)  [unwired: 4 in, 4 out]
        n187 = in-place-cluster #25("FP.VI Tree Value"="", "FP.Selected VI Data"=-1, "FP Refs.VI Tree"=w387) -> (w383:T1)
      }
    }
  }
  "State Data out" <- w5
  "error out" <- w1
